vi "Set Results.vi"(8 "error in (no error)":errorcluster, 10 "Results":variant, 11 "Abstract Results Msg in":refnum<class "Abstract Results Msg.lvclass">) -> (0 "error out":errorcluster, 3 "Abstract Results Msg out":refnum<class "Abstract Results Msg.lvclass">)   [LabVIEW 2013, in "Hot And Cold Source Unit Model.lvlib" / "Abstract Results Msg.lvclass"]
uses:
  Abstract Results Msg.lvclass
  Abstract Results Msg.lvclass/Abstract Results Msg.ctl
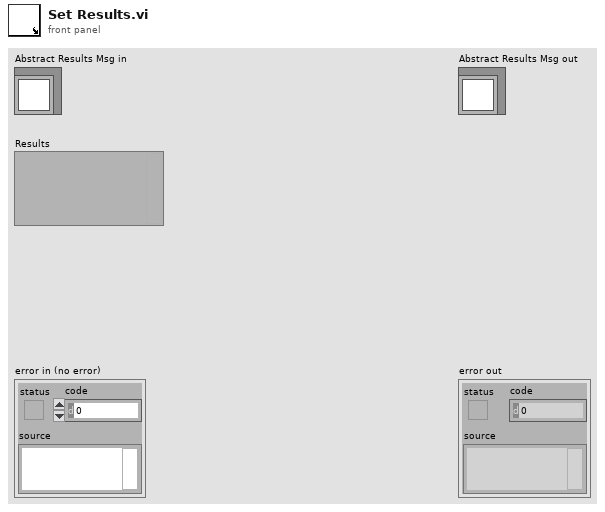
[diagram p1: front panel]
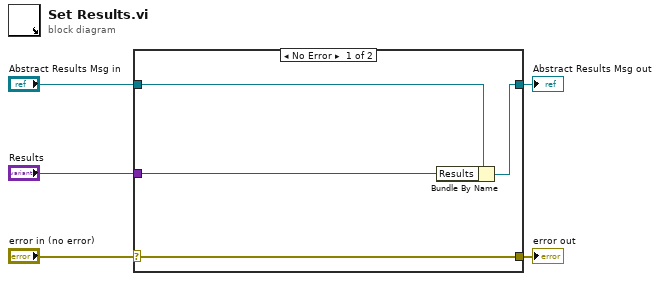
[diagram p0: block diagram]
diagram:
  n1 = case shown="No Error" "error in (no error)" {
    selector: "error in (no error)" -> [w9 w10]
    tunnel: [w9 w10] -> w4
    tunnel: [w7 w11] -> w2
    tunnel: "Abstract Results Msg in" -> [w8 w11]
    tunnel: "Results" -> [w6 _]
    frame No Error {
      n2 = Bundle By Name(cluster=w8, "Results"=w6) -> (w7:refnum<class "Abstract Results Msg.lvclass">)
    }
    frame Error {
    }
  }
  "error out" <- w4
  "Abstract Results Msg out" <- w2
